vi "Init Global Log.vi"(7 "Application Log in":refnum<class "Application Log.lvclass">, 8 "error in (no error)":errorcluster, 9 "iType":string, 10 "iName":string) -> (0 "error out":errorcluster)   [LabVIEW 2016, in "Stream Log.lvlib" / "Global Application Log.lvclass"]
doc: "--\nCopyright © 2017 Composed SystemsI All rights reserved.\n\nAuthor: Jon McBee <jon.mcbee@composed.io>\n\nThis library is provided \"AS IS\" ,WITHOUT WARRANTIES OR\nCONDITIONS OF ANY KIND, either express or implied.\n\nComposed Systems -- composed.io\n\nStream 0.0.1.1\nJon McBee - Composed Systems\nCopyright (c) 2017, Composed Systems"
uses:
  <userlib>/Composed Systems/Stream/Log/Global Application Log/Global Application Log.lvclass
  <userlib>/Composed Systems/Stream/Log/Application Log/Application Log.lvclass
  <userlib>/Composed Systems/Stream/Log/Global Application Log/Log Reference Action.ctl
  <userlib>/Composed Systems/Stream/Log/Application Log/Log Level.ctl
  <userlib>/Composed Systems/Stream/Log/Global Application Log/Global Application Log.lvclass/Global Application Log.ctl
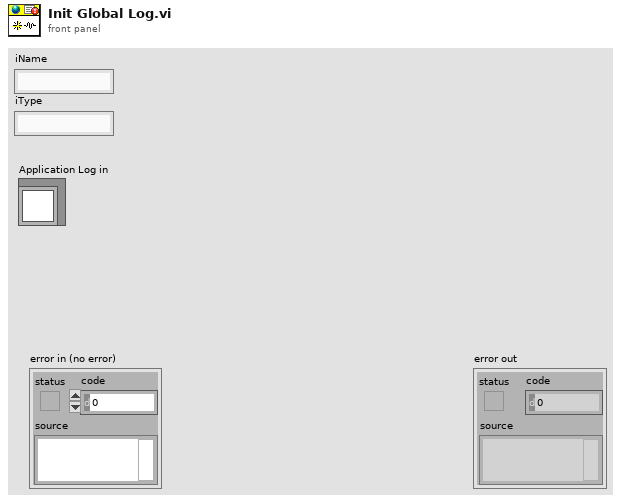
[diagram p1: front panel]
types:
  T1 = typedef "Stream Log.lvlib/Application Log.lvclass/Log Level.ctl" = enum16{"Imperative", "Major", "Minor", "Debug", "Off"}
  T2 = typedef "Stream Log.lvlib/Global Application Log.lvclass/Log Reference Action.ctl" = enum16{"Get Log Reference", "Set Log Reference"}
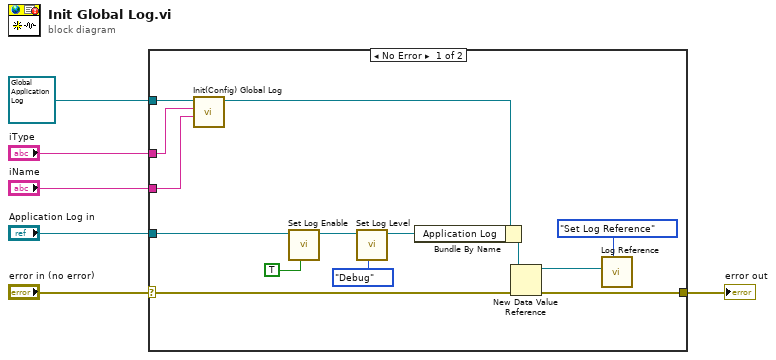
[diagram p0: block diagram]
diagram:
  n1 = case shown="No Error" "error in (no error)" {
    selector: "error in (no error)" -> [w18 w21]
    tunnel: [w17 w21] -> w5
    tunnel: refnum<class "Global Application Log.lvclass"> refnum ("Global Application Log in") -> [w16 _]
    tunnel: "iType" -> [w15 _]
    tunnel: "iName" -> [w14 _]
    tunnel: "Application Log in" -> [w7 _]
    frame No Error {
      n2 = call <userlib>:"Init(Config) Global Log.vi"("iName"=w14, "iType"=w15, "Global Application Log in"=w16) -> ("Global Application Log out"=w13:refnum<class "Global Application Log.lvclass">)  [unwired: 7 in, 1 out]
      n3 = call <userlib>:"Set Log Enable.vi"("Configuration.Enabled"=TRUE, "Application Log in"=w7) -> ("Application Log out"=w11:refnum<class "Application Log.lvclass">)  [unwired: 8 in, 1 out]
      n4 = call <userlib>:"Set Log Level.vi"("Configuration.Level"=Log_Level."Debug", "Application Log in"=w11) -> ("Application Log out"=w10:refnum<class "Application Log.lvclass">)  [unwired: 8 in, 1 out]
      n5 = Bundle By Name(cluster=w13, "Application Log"=w10) -> (w12:refnum<class "Global Application Log.lvclass">)
      n6 = New Data Value Reference(data value=w12, error in=w18) -> (data value reference=w19:refnum<data-value>, error out=w17:errorcluster)
      n7 = call <userlib>:"Log Reference.vi"("Action"=Log_Reference_Action."Set Log Reference", "Global Log Reference"=w19) -> ()  [unwired: 9 in, 1 out]
    }
    frame Error {
    }
  }
  "error out" <- w5
